vi "DIN Logic FPGA (SubVI).vi"(0 "DIO Module":u8, 5 "Masks":T1={"DIN1 Mask Out1"=[FALSE, FALSE, FALSE, FALSE, FALSE, FALSE, FALSE, FALSE], "DIN1 Mask Out2"=[FALSE, FALSE, FALSE, FALSE, FALSE, FALSE, FALSE, FALSE], "DIN1 Mask Out3"=[FALSE, FALSE, FALSE, FALSE, FALSE, FALSE, FALSE, FALSE], "DIN1 Mask Out4"=[FALSE, FALSE, FALSE, FALSE, FALSE, FALSE, FALSE, FALSE]}) -> (8 "DIN Triggered Out":cluster{bool, bool, bool, bool}, 10 "DIN TrigMask Out":bool[](array[boolean]))   [LabVIEW 2014]
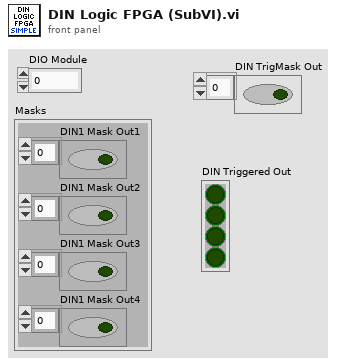
[diagram p1: front panel]
types:
  T1 = cluster{"DIN1 Mask Out1":bool[], "DIN1 Mask Out2":bool[], "DIN1 Mask Out3":bool[], "DIN1 Mask Out4":bool[]}
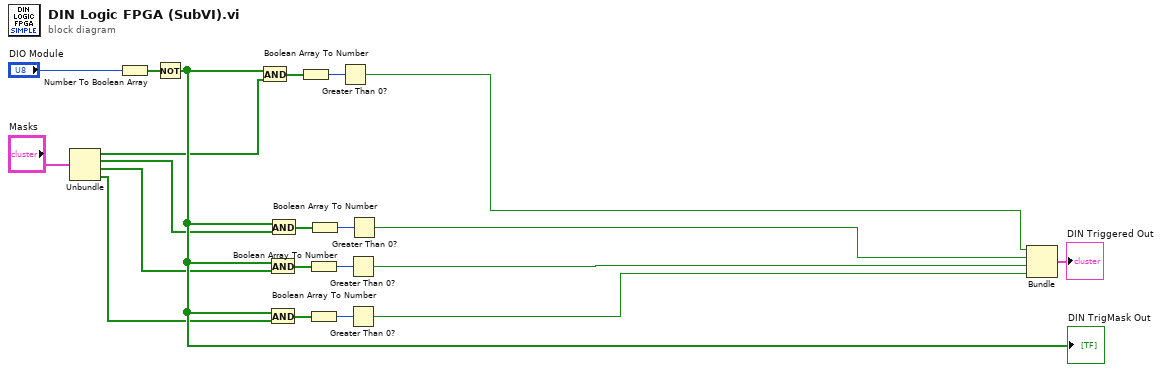
[diagram p0: block diagram]
diagram:
  n1 = Unbundle("Masks") -> ("DIN1 Mask Out1"=w9:bool[], "DIN1 Mask Out2"=w8:bool[], "DIN1 Mask Out3"=w7:bool[], "DIN1 Mask Out4"=w6:bool[])
  n2 = Number To Boolean Array(number="DIO Module") -> (Boolean array=w19:bool[])
  n3 = Not(x=w19) -> (.not. x?=w10:bool[])
  "DIN TrigMask Out" <- w10
  n4 = And(x=w10, y=w9) -> (x .and. y?=w18:bool[])
  n5 = And(x=w10, y=w7) -> (x .and. y?=w14:bool[])
  n6 = And(x=w10, y=w6) -> (x .and. y?=w12:bool[])
  n7 = And(x=w10, y=w8) -> (x .and. y?=w13:bool[])
  n8 = Boolean Array To Number(Boolean array=w18) -> (number=w20:u8)
  n9 = Boolean Array To Number(Boolean array=w14) -> (number=w15:u8)
  n10 = Boolean Array To Number(Boolean array=w12) -> (number=w11:u8)
  n11 = Boolean Array To Number(Boolean array=w13) -> (number=w16:u8)
  n12 = Greater Than 0?(x=w20) -> (x > 0?=w5:bool)
  n13 = Greater Than 0?(x=w15) -> (x > 0?=w2:bool)
  n14 = Greater Than 0?(x=w11) -> (x > 0?=w3:bool)
  n15 = Greater Than 0?(x=w16) -> (x > 0?=w1:bool)
  n16 = Bundle(w5, w1, w2, w3) -> (→"DIN Triggered Out":cluster{bool, bool, bool, bool})  [unwired: 1 in]
